vi "CurrentCorrection.vi"(8 "Calib_data":u8[](array[numeric]) format="%02x", 11 "Current_in_mA":u16[](array[numeric])) -> (2 "Correct_Code":u16[](array[numeric]) format="%03x")   [LabVIEW 2015]
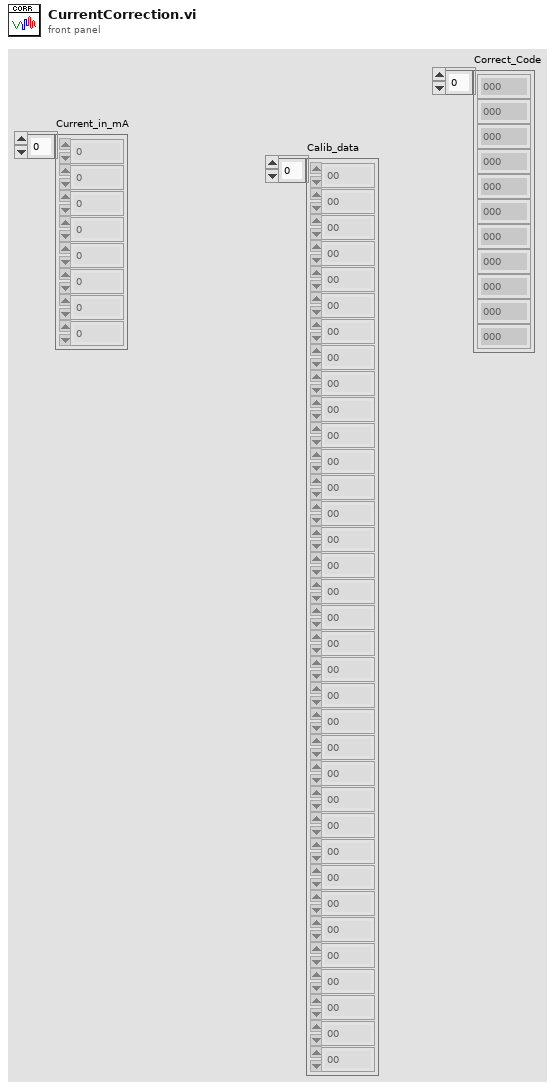
[diagram p1: front panel]
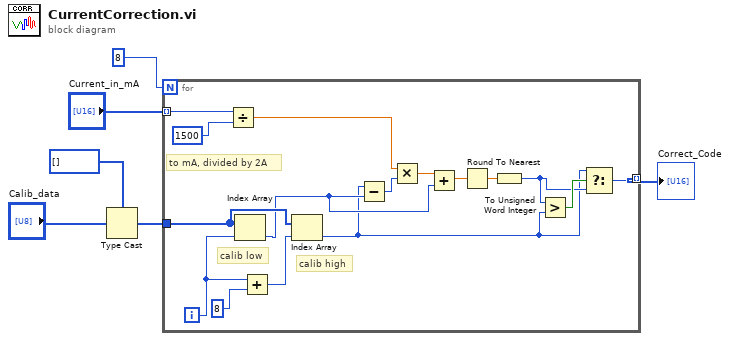
[diagram p0: block diagram]
diagram:
  n1 = Type Cast(type=u16[] [], x="Calib_data") -> (*(type *) &x=w3:u16[])
  n2 = for {
    N: 8 -> [_]
    tunnel: w3 -> [w21]
    tunnel: "Current_in_mA" -> [w18] mode=indexing
    tunnel: [w8] -> w1 mode=indexing
    i -> [w20]
    # "to mA, divided by 2A"
    # "calib high"
    # "calib low"
    n3 = Divide(x=w18, y=u16 1500) -> (x/y=w15:dbl)
    n4 = Index Array(array=w21, index=w20) -> (element=w13:u16)
    n5 = Add(x=w20, y=8) -> (x+y=w19:i32)
    n6 = Index Array(array=w21, index=w19) -> (element=w7:u16)
    n7 = Subtract(x=w7, y=w13) -> (x-y=w16:u16)
    n8 = Multiply(x=w15, y=w16) -> (x*y=w14:dbl)
    n9 = Add(x=w14, y=w13) -> (x+y=w12:dbl)
    n10 = Round To Nearest(number=w12) -> (nearest integer value=w11:dbl)
    n11 = To Unsigned Word Integer(number=w11) -> (unsigned 16bit integer=w9:u16)
    n12 = Greater?(x=w9, y=w7) -> (0:w10:bool)
    n13 = Select(t=w7, s=w10, f=w9) -> (s? t:f=w8:u16)
  }
  "Correct_Code" <- w1
